vi "IMU_test.vi"(8 "Data Type":u16(ring)=1 items=["Uncorrected (gyro drift)", "Corrected"], 9 "Print Out Type":u16(ring)=1 items=["Raw", "Euler"], 11 "Connection":refnum<k16>) -> (1 "Ouput Size":i32, 2 "Output":sgl[](array[numeric]))   [LabVIEW 2012]
panel:
  out "error out":errorcluster
  out "Raw Data":u8[](array[numeric])
  # "Arduino is setup to send data to 10.8.36.2 on port 22"
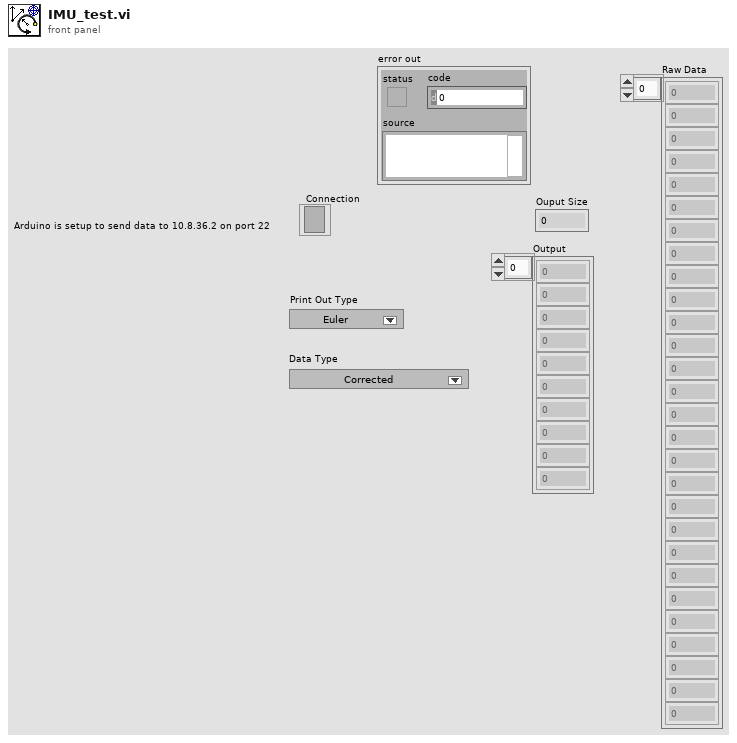
[diagram p1: front panel]
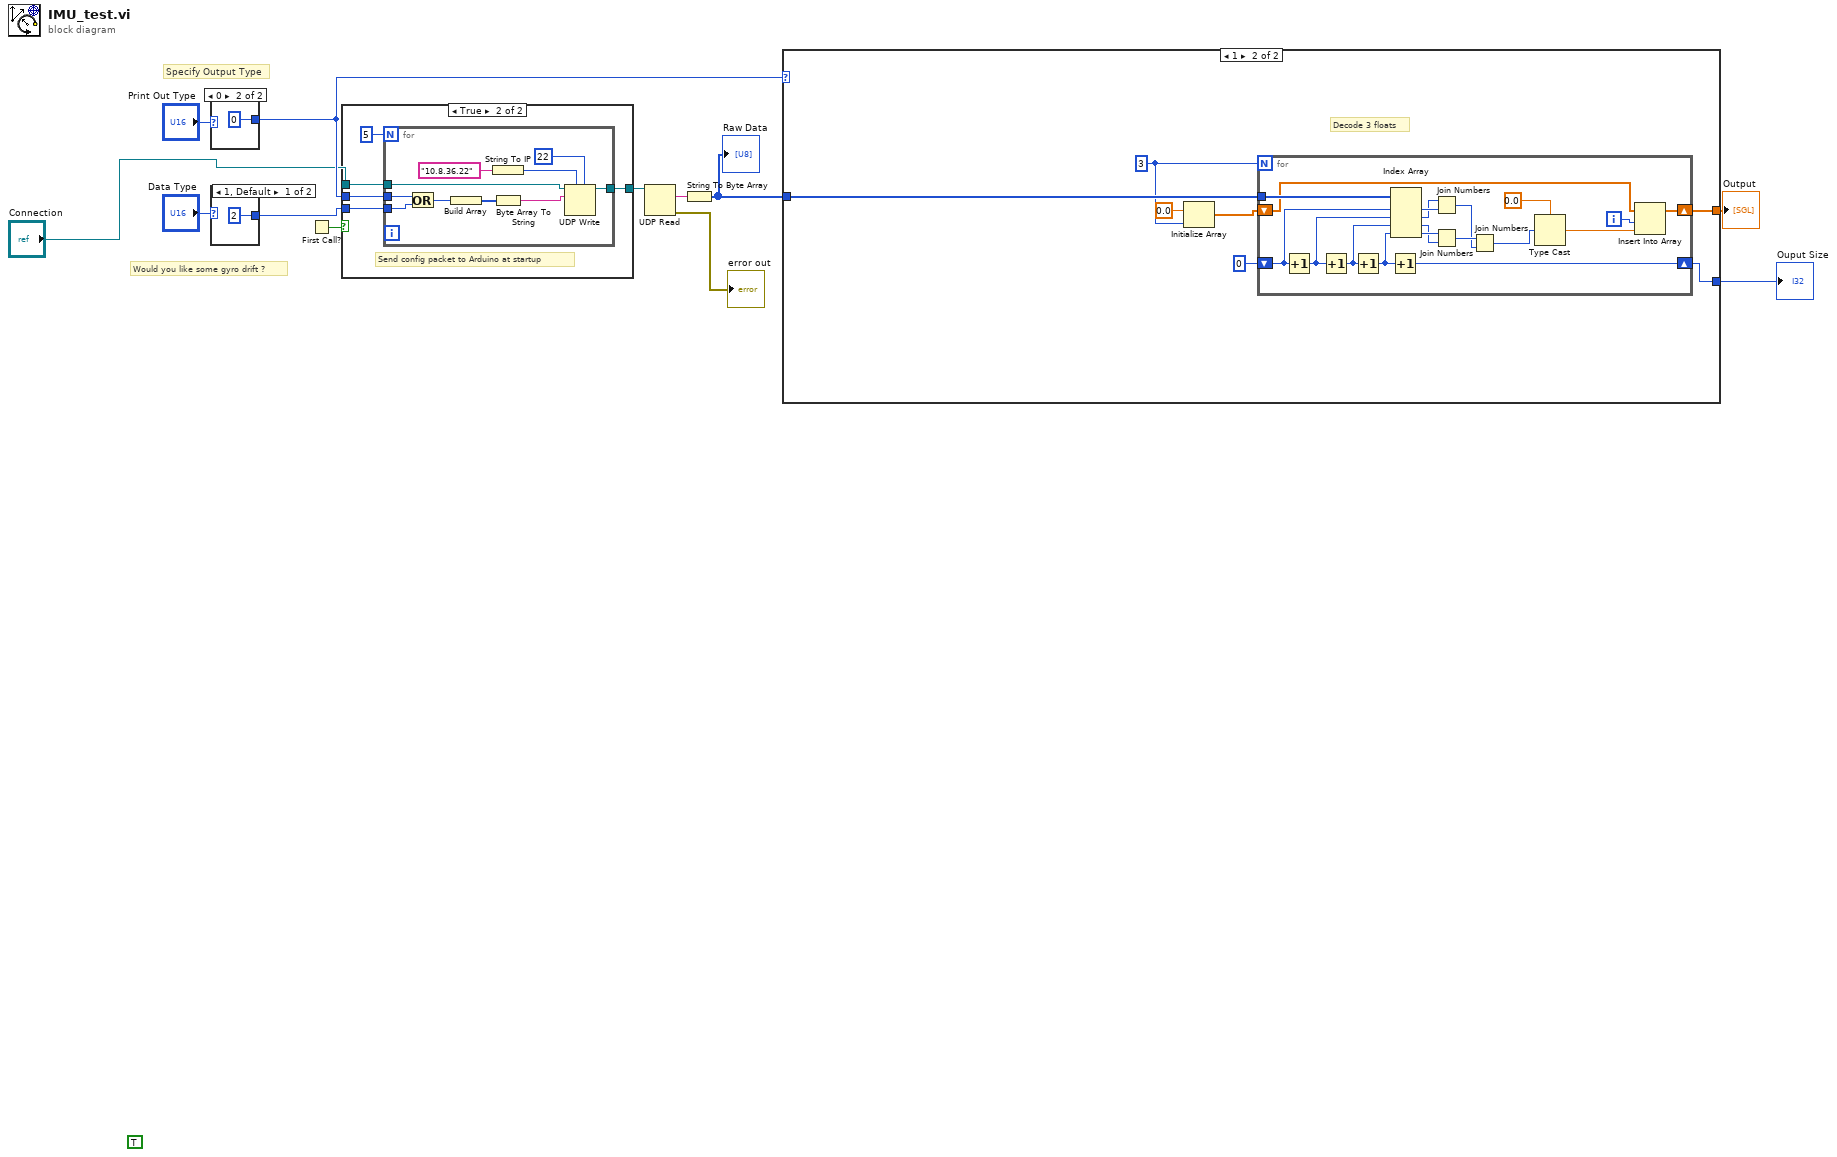
[diagram p0: block diagram]
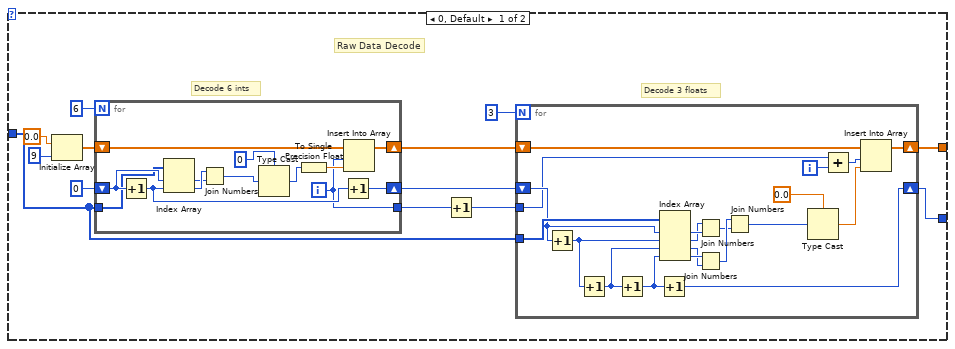
[diagram p2: hidden frame]
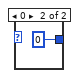
[diagram p4: hidden frame]
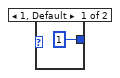
[diagram p5: hidden frame]
diagram:
  (unwired) TRUE
  # "Would you like some gyro drift ?"
  # "Specify Output Type"
  n1 = case shown="0" "Print Out Type" {
    tunnel: [u8 1 u8 0] -> w7
    frame 1, Default {
    }
    frame 0 {
    }
  }
  n2 = case shown="1, Default" "Data Type" {
    tunnel: [u8 2 u8 0] -> w9
    frame 1, Default {
    }
    frame 0 {
    }
  }
  n3 = First Call?() -> (First Call?: T/F=w8:bool)
  n4 = case shown="True" w8 {
    tunnel: w7 -> [_ w22]
    tunnel: w9 -> [_ w21]
    tunnel: [w17 w19] -> w6
    tunnel: "Connection" -> [w17 w18]
    frame False {
    }
    frame True {
      # "Send config packet to Arduino at startup"
      n5 = for {
        N: 5 -> [_]
        tunnel: w22 -> [w32]
        tunnel: w21 -> [w31]
        tunnel: [w24] -> w19
        tunnel: w18 -> [w23]
        n6 = Or(x=w32, y=w31) -> (x .or. y?=w29:u8)
        n7 = Build Array(w29) -> (w28:u8[])
        n8 = String To IP(1:"10.8.36.22") -> (0:w26:u32)
        n9 = Byte Array To String(unsigned byte array=w28) -> (string=w30:string)
        n10 = UDP Write(address=w26, port or service name=u16 22, connection ID=w23, data in=w30) -> (3:w24:refnum<k16>)  [unwired: 2 in, 1 out]
      }
    }
  }
  n11 = UDP Read(connection ID=w6) -> (data out=w5:string, error out=→"error out":errorcluster)  [unwired: 3 in, 3 out]
  n12 = String To Byte Array(string=w5) -> (unsigned byte array=w4:u8[])
  "Raw Data" <- w4
  n13 = case shown="1" w7 {
    tunnel: w4 -> [w36 w85]
    tunnel: [w37 w80] -> w10
    tunnel: [w33 w79] -> w2
    frame 0, Default {
      # "Decode 3 floats"
      # "Decode 6 ints"
      # "Raw Data Decode"
      n14 = Initialize Array(sgl 0.0, 9) -> (w41:sgl[])
      n15 = for {
        N: 6 -> [_]
        shift-right: [w74] -> w39
        shift-left: 0 -> [w75]
        shift-right: [w76] -> w38
        shift-left: w41 -> [w73]
        tunnel: w36 -> [w72]
        tunnel: [w66] -> w35
        i -> [w66]
        n16 = Increment(x=w75) -> (x+1=w71:i32)
        n17 = Index Array(array=w72, index #1=w75, index #2=w71) -> (element #1=w69:u8, element #2=w70:u8)
        n18 = Join Numbers(hi=w70, lo=w69) -> ((hi.lo)=w77:u16)
        n19 = Type Cast(type=i16 0, x=w77) -> (*(type *) &x=w68:i16)
        n20 = To Single Precision Float(number=w68) -> (single precision float=w67:sgl)
        n21 = Increment(x=w71) -> (x+1=w74:i32)
        n22 = Insert Into Array(array=w73, index=w66, new element=w67) -> (w76:sgl[])
      }
      n23 = Increment(x=w35) -> (x+1=w34:i32)
      n24 = for {
        N: 3 -> [_]
        tunnel: w36 -> [w63]
        shift-right: [w50] -> w33
        shift-left: w39 -> [w52]
        shift-right: [w53] -> w37
        shift-left: w38 -> [w49]
        tunnel: w34 -> [w47]
        i -> [w48]
        n25 = Increment(x=w52) -> (x+1=w58:i32)
        n26 = Increment(x=w58) -> (x+1=w57:i32)
        n27 = Increment(x=w57) -> (x+1=w51:i32)
        n28 = Increment(x=w51) -> (x+1=w50:i32)
        n29 = Index Array(array=w63, index #1=w52, index #2=w58, index #3=w57, index #4=w51) -> (element #1=w62:u8, element #2=w61:u8, element #3=w59:u8, element #4=w60:u8)
        n30 = Join Numbers(hi=w61, lo=w62) -> ((hi.lo)=w64:u16)
        n31 = Join Numbers(hi=w60, lo=w59) -> ((hi.lo)=w65:u16)
        n32 = Join Numbers(hi=w65, lo=w64) -> ((hi.lo)=w55:u32)
        n33 = Type Cast(type=sgl 0.0, x=w55) -> (*(type *) &x=w54:sgl)
        n34 = Add(x=w47, y=w48) -> (x+y=w46:i32)
        n35 = Insert Into Array(array=w49, index=w46, new element=w54) -> (w53:sgl[])
      }
    }
    frame 1 {
      w82 = 3
      # "Decode 3 floats"
      n36 = Initialize Array(sgl 0.0, w82) -> (w81:sgl[])
      n37 = for {
        N: w82 -> [_]
        tunnel: w85 -> [w101]
        shift-right: [w87] -> w79
        shift-left: 0 -> [w90]
        shift-right: [w91] -> w80
        shift-left: w81 -> [w86]
        i -> [w89]
        n38 = Increment(x=w90) -> (x+1=w96:i32)
        n39 = Increment(x=w96) -> (x+1=w95:i32)
        n40 = Increment(x=w95) -> (x+1=w88:i32)
        n41 = Increment(x=w88) -> (x+1=w87:i32)
        n42 = Index Array(array=w101, index #1=w90, index #2=w96, index #3=w95, index #4=w88) -> (element #1=w100:u8, element #2=w99:u8, element #3=w97:u8, element #4=w98:u8)
        n43 = Join Numbers(hi=w99, lo=w100) -> ((hi.lo)=w102:u16)
        n44 = Join Numbers(hi=w98, lo=w97) -> ((hi.lo)=w103:u16)
        n45 = Join Numbers(hi=w103, lo=w102) -> ((hi.lo)=w93:u32)
        n46 = Type Cast(type=sgl 0.0, x=w93) -> (*(type *) &x=w92:sgl)
        n47 = Insert Into Array(array=w86, index=w89, new element=w92) -> (w91:sgl[])
      }
    }
  }
  "Output" <- w10
  "Ouput Size" <- w2
